vi "Configure RunTime Path.vi"(1 "Input Path":path) -> (0 "Updated Path":path)   [LabVIEW 2019, in "TSC File IO.lvlib"]
doc: "This VI will convert the input file path to remove the lvlibp namespace if it is in the path.\n\nInputs:\n-Input Path [path] - the starting path\n\nOutputs:\n-Updated Path [path] - the updated path; if the VI is not in a packed library, this will be left alone, however if the VI is in a packed library strip off the extra path info\n\n<b>Code Developed By:</b>\nDaniel Coons\nTechnology Service Corporation\n1983 S Liberty Drive\nBloomington, IN 47403\nwww.tsc.com\\atcs"
uses:
  TSC File IO.lvlib
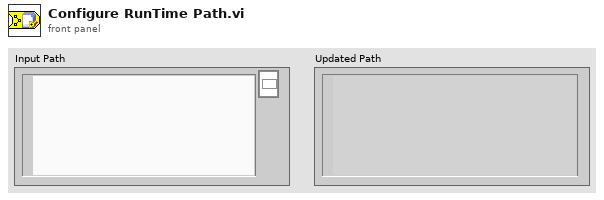
[diagram p1: front panel]
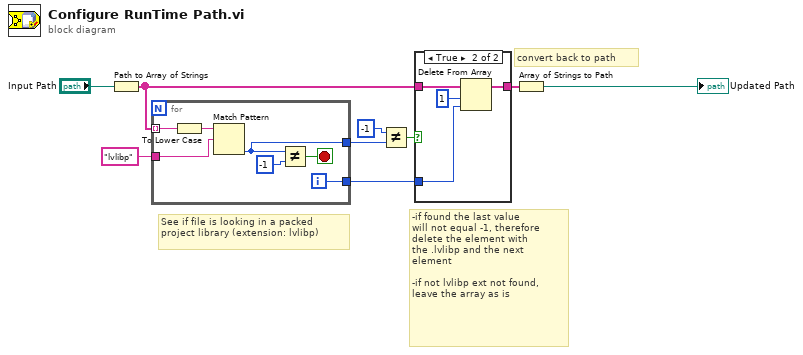
[diagram p0: block diagram]
diagram:
  # "convert back to path"
  # "-if found the last value\nwill not equal -1, therefore\ndelete the element with\nthe .lvlibp and the next\nelement\n\n-if not lvlibp ext not found,\nleave the array as is"
  # "See if file is looking in a packed\nproject library (extension: lvlibp)"
  n1 = Path to Array of Strings(0:"Input Path") -> (2:w2:string[])  [unwired: 1 out]
  n2 = for {
    tunnel: w2 -> [w16] mode=indexing
    tunnel: "lvlibp" ("element") -> [w14]
    tunnel: [w13] -> w3
    tunnel: [w10] -> w4
    i -> [w13]
    stop <- w11 stop-if-true
    n3 = To Lower Case(string=w16) -> (all lower case string=w15:string)
    n4 = Match Pattern(string=w15, regular expression=w14) -> (offset past match=w10:i32)  [unwired: 1 in, 3 out]
    n5 = Not Equal?(x=w10, y=-1) -> (x != y?=w11:bool)
  }
  n6 = Not Equal?(x=-1 ("y"), y=w4) -> (x != y?=w6:bool)
  n7 = case shown="True" w6 {
    tunnel: w2 -> [w17 w21]
    tunnel: w3 -> [_ w20]
    tunnel: [w17 w18] -> w7
    frame False {
    }
    frame True {
      n8 = Delete From Array(array=w21, length=1, index=w20) -> (array with subset deleted=w18:string[])  [unwired: 1 out]
    }
  }
  n9 = Array of Strings to Path(0:w7) -> (2:→"Updated Path":path)  [unwired: 1 in]
